vi "Graph_Extras.vi"(8 "Scope+Safety":T3={"Safety First"={"lim reset"=FALSE, "no limit"=FALSE, "pos slew rate * dt"=100, "neg slew rate * dt"=-100, "Count(Ticks)"=0}, "Scope IPs"={"Trigger Direction"=enum."minus-plus", "Trigger Delay (ms)"=0.0, "Aquisition Rate (kHz)"=4000.0, "Trigger Offset (V)"=0.0, "Scale Offset"={"Scaling"={"Error signal"=1, "Output"=1, "DC Monitor"=1, "Threshold"=1}, "Offset"={"Error Signal"=0, "Output"=0, "DC Monitor"=0, "Threshold"=0}}}}, 11 "Graph Extras":T4={"Error Bit Sh."={"パラメ A"=0, "パラメ B"=0, "EPR BS"=0, "Graph BS"=0, "HD A x"=0, "HD A p"=0, "HD B x"=0, "HD B p"=0}, "I Max value"=20000, "I2 Max value"=20000, "Scan Offset"={"パラメ A"=0.0, "パラメ B"=0.0, "EPR BS"=0.0, "Graph BS"=0.0, "HD A"=0.0, "HD B"=0.0}, "Scan Ampl."={"パラメ A"=0.0, "パラメ B"=0.0, "EPR BS"=0.0, "Graph BS"=0.0, "HD A"=0.0, "HD B"=0.0}, "Scan-PII thresh"={"パラメ A"=1000, "パラメ B"=1000, "EPR BS"=1000, "Graph BS"=1000, "Homodyne A"=0, "Homodyne B"=0}, "Re-Scan thresh"={"パラメ A"=0, "パラメ B"=0, "EPR BS"=0, "Graph BS"=0, "Homodyne A"=0, "Homodyne B"=0}, "Post-Offset"={"HD A x"=0.0, "HD A p"=0.0, "HD B x"=0.0, "HD B p"=0.0}}) -> (0 "Extras Homodyne B":T1, 1 "Extras Homodyne A":T1, 2 "Extras Graph":T2, 3 "Extras EPR BS":T2, 5 "Extras パラメ B":T2, 7 "Extras パラメ A":T2)   [LabVIEW 2010]
uses:
  Strict Type Defs/Graph Extras.ctl
  Strict Type Defs/Double Graph control.ctl
  Strict Type Defs/I16 Graph Control.ctl
  Strict Type Defs/Scope and Safety.ctl
  Strict Type Defs/Extras PII Graph.ctl
  Strict Type Defs/Extras PII Graph HD.ctl
panel:
  in  "Extras HD":T1
  in  "Extras PII Graph":T2
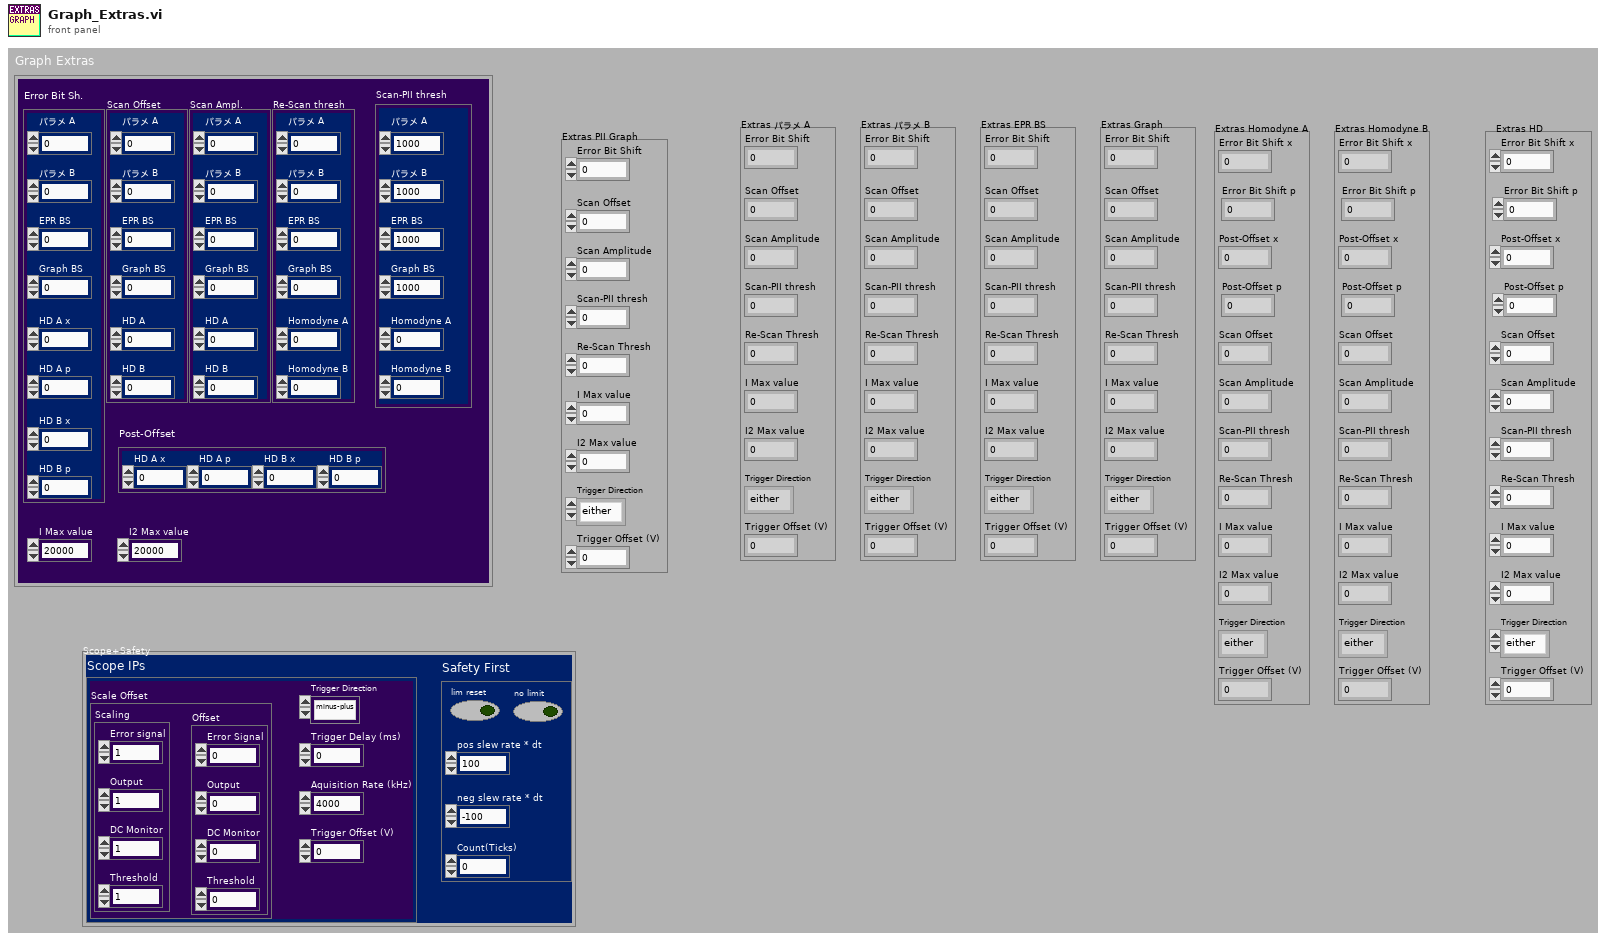
[diagram p1: front panel]
types:
  T1 = typedef "Extras PII Graph HD.ctl" = cluster{"Error Bit Shift p":i16, "Scan Offset":dbl, "Scan Amplitude":dbl, "Scan-PII thresh":i16, "Re-Scan Thresh":i16, "I Max value":i32, "I2 Max value":i32, "Trigger Direction":enum8{"either", "minus-plus", "plus-minus"}, "Trigger Offset (V)":dbl, "Error Bit Shift x":i16, "Post-Offset p":dbl, "Post-Offset x":dbl}
  T2 = typedef "Extras PII Graph.ctl" = cluster{"Error Bit Shift":i16, "Scan Offset":dbl, "Scan Amplitude":dbl, "Scan-PII thresh":i16, "Re-Scan Thresh":i16, "I Max value":i32, "I2 Max value":i32, "Trigger Direction":enum8{"either", "minus-plus", "plus-minus"}, "Trigger Offset (V)":dbl}
  T3 = typedef "Scope and Safety.ctl" = cluster{"Safety First":cluster{"lim reset":bool, "no limit":bool, "pos slew rate * dt":i16, "neg slew rate * dt":i16, "Count(Ticks)":u32}, "Scope IPs":cluster{"Trigger Direction":enum8{"either", "minus-plus", "plus-minus"}, "Trigger Delay (ms)":dbl, "Aquisition Rate (kHz)":dbl, "Trigger Offset (V)":dbl, "Scale Offset":cluster{"Scaling":cluster{"Error signal":i16, "Output":i16, "DC Monitor":i16, "Threshold":i16}, "Offset":cluster{"Error Signal":i16, "Output":i16, "DC Monitor":i16, "Threshold":i16}}}}
  T4 = typedef "Graph Extras.ctl" = cluster{"Error Bit Sh.":cluster{"パラメ A":i16, "パラメ B":i16, "EPR BS":i16, "Graph BS":i16, "HD A x":i16, "HD A p":i16, "HD B x":i16, "HD B p":i16}, "I Max value":i32, "I2 Max value":i32, "Scan Offset":T5, "Scan Ampl.":T5, "Scan-PII thresh":T6, "Re-Scan thresh":T6, "Post-Offset":cluster{"HD A x":dbl, "HD A p":dbl, "HD B x":dbl, "HD B p":dbl}}
  T5 = typedef "Double Graph control.ctl" = cluster{"パラメ A":dbl, "パラメ B":dbl, "EPR BS":dbl, "Graph BS":dbl, "HD A":dbl, "HD B":dbl}
  T6 = typedef "I16 Graph Control.ctl" = cluster{"パラメ A":i16, "パラメ B":i16, "EPR BS":i16, "Graph BS":i16, "Homodyne A":i16, "Homodyne B":i16}
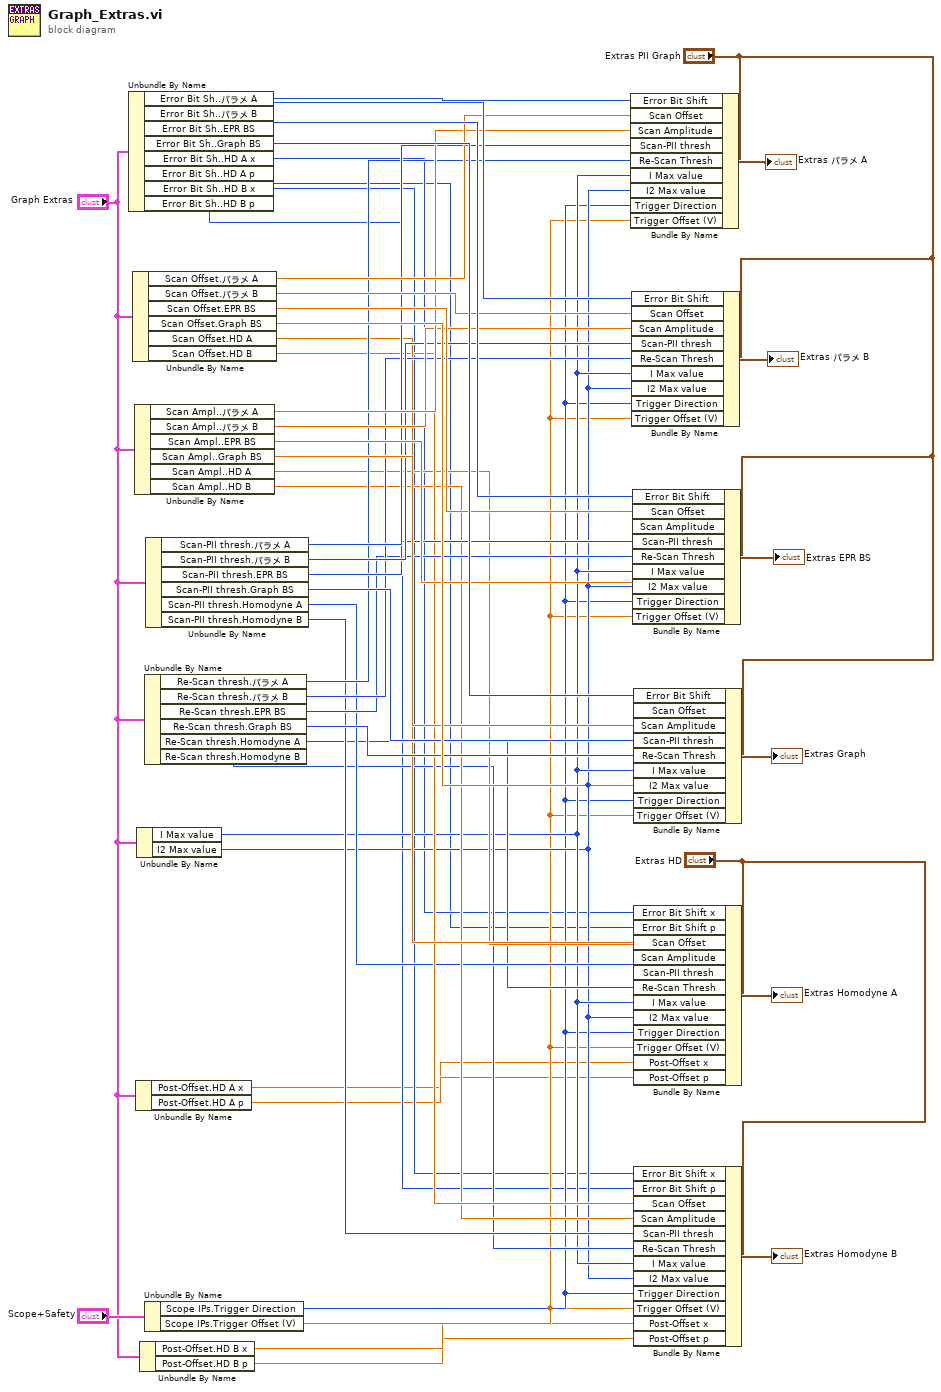
[diagram p0: block diagram]
diagram:
  n1 = Unbundle By Name("Graph Extras") -> ("Error Bit Sh..パラメ A"=w45:i16, "Error Bit Sh..パラメ B"=w44:i16, "Error Bit Sh..EPR BS"=w43:i16, "Error Bit Sh..Graph BS"=w42:i16, "Error Bit Sh..HD A x"=w9:i16, "Error Bit Sh..HD A p"=w8:i16, "Error Bit Sh..HD B x"=w7:i16, "Error Bit Sh..HD B p"=w6:i16)
  n2 = Unbundle By Name("Graph Extras") -> ("Scan Offset.パラメ A"=w41:dbl, "Scan Offset.パラメ B"=w40:dbl, "Scan Offset.EPR BS"=w39:dbl, "Scan Offset.Graph BS"=w38:dbl, "Scan Offset.HD A"=w22:dbl, "Scan Offset.HD B"=w21:dbl)
  n3 = Unbundle By Name("Graph Extras") -> ("Scan Ampl..パラメ A"=w37:dbl, "Scan Ampl..パラメ B"=w36:dbl, "Scan Ampl..EPR BS"=w35:dbl, "Scan Ampl..Graph BS"=w34:dbl, "Scan Ampl..HD A"=w20:dbl, "Scan Ampl..HD B"=w19:dbl)
  n4 = Unbundle By Name("Graph Extras") -> ("Post-Offset.HD A x"=w4:dbl, "Post-Offset.HD A p"=w5:dbl)
  n5 = Unbundle By Name("Graph Extras") -> ("I Max value"=w14:i32, "I2 Max value"=w13:i32)
  n6 = Unbundle By Name("Graph Extras") -> ("Post-Offset.HD B x"=w2:dbl, "Post-Offset.HD B p"=w1:dbl)
  n7 = Unbundle By Name("Graph Extras") -> ("Re-Scan thresh.パラメ A"=w29:i16, "Re-Scan thresh.パラメ B"=w28:i16, "Re-Scan thresh.EPR BS"=w27:i16, "Re-Scan thresh.Graph BS"=w26:i16, "Re-Scan thresh.Homodyne A"=w16:i16, "Re-Scan thresh.Homodyne B"=w15:i16)
  n8 = Unbundle By Name("Scope+Safety") -> ("Scope IPs.Trigger Direction"=w12:enum8{"either", "minus-plus", "plus-minus"}, "Scope IPs.Trigger Offset (V)"=w11:dbl)
  n9 = Unbundle By Name("Graph Extras") -> ("Scan-PII thresh.パラメ A"=w33:i16, "Scan-PII thresh.パラメ B"=w32:i16, "Scan-PII thresh.EPR BS"=w31:i16, "Scan-PII thresh.Graph BS"=w30:i16, "Scan-PII thresh.Homodyne A"=w18:i16, "Scan-PII thresh.Homodyne B"=w17:i16)
  n10 = Bundle By Name(cluster="Extras PII Graph", "Error Bit Shift"=w45, "Scan Offset"=w41, "Scan Amplitude"=w37, "Scan-PII thresh"=w33, "Re-Scan Thresh"=w29, "I Max value"=w14, "I2 Max value"=w13, "Trigger Direction"=w12, "Trigger Offset (V)"=w11) -> (→"Extras パラメ A":T2)
  n11 = Bundle By Name(cluster="Extras PII Graph", "Error Bit Shift"=w44, "Scan Offset"=w40, "Scan Amplitude"=w36, "Scan-PII thresh"=w32, "Re-Scan Thresh"=w28, "I Max value"=w14, "I2 Max value"=w13, "Trigger Direction"=w12, "Trigger Offset (V)"=w11) -> (→"Extras パラメ B":T2)
  n12 = Bundle By Name(cluster="Extras PII Graph", "Error Bit Shift"=w43, "Scan Offset"=w39, "Scan Amplitude"=w35, "Scan-PII thresh"=w31, "Re-Scan Thresh"=w27, "I Max value"=w14, "I2 Max value"=w13, "Trigger Direction"=w12, "Trigger Offset (V)"=w11) -> (→"Extras EPR BS":T2)
  n13 = Bundle By Name(cluster="Extras PII Graph", "Error Bit Shift"=w42, "Scan Offset"=w38, "Scan Amplitude"=w34, "Scan-PII thresh"=w30, "Re-Scan Thresh"=w26, "I Max value"=w14, "I2 Max value"=w13, "Trigger Direction"=w12, "Trigger Offset (V)"=w11) -> (→"Extras Graph":T2)
  n14 = Bundle By Name(cluster="Extras HD", "Error Bit Shift x"=w9, "Error Bit Shift p"=w8, "Scan Offset"=w22, "Scan Amplitude"=w20, "Scan-PII thresh"=w18, "Re-Scan Thresh"=w16, "I Max value"=w14, "I2 Max value"=w13, "Trigger Direction"=w12, "Trigger Offset (V)"=w11, "Post-Offset x"=w4, "Post-Offset p"=w5) -> (→"Extras Homodyne A":T1)
  n15 = Bundle By Name(cluster="Extras HD", "Error Bit Shift x"=w7, "Error Bit Shift p"=w6, "Scan Offset"=w21, "Scan Amplitude"=w19, "Scan-PII thresh"=w17, "Re-Scan Thresh"=w15, "I Max value"=w14, "I2 Max value"=w13, "Trigger Direction"=w12, "Trigger Offset (V)"=w11, "Post-Offset x"=w2, "Post-Offset p"=w1) -> (→"Extras Homodyne B":T1)
